vi "HW Display Loop Processor.vi"(4 "error in (no error)":errorcluster) -> (0 "error out":errorcluster, 1 "Tx Stat":T1, 2 "TxPower":dbl[](array[numeric]) format="%.2f", 3 "TxOn":bool[](array[boolean]))   [LabVIEW 2011]
uses:
  API/Controls/PIM.API.Command.Unique.ctl
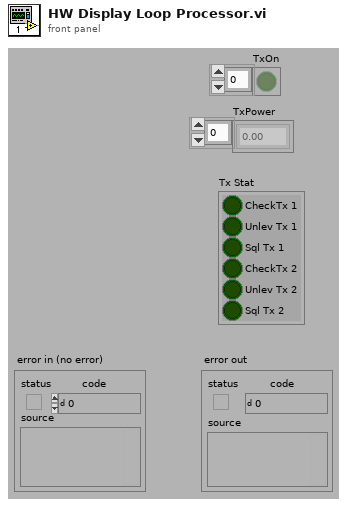
[diagram p1: front panel]
types:
  T1 = cluster{"CheckTx 1":bool, "Unlev Tx 1":bool, "Sql Tx 1":bool, "CheckTx 2":bool, "Unlev Tx 2":bool, "Sql Tx 2":bool}
  T2 = typedef "PIM.API.Command.Unique.ctl" = cluster{"#attributes":cluster{"Action":string}, "Double":dbl[], "Integer":i32[], "Boolean":bool[], "String":string[]}
  T3 = typedef "PIM.API.Response.Unique.ctl" = cluster{"#attributes":cluster{"Action":string, "Units":string}, "Double":dbl[], "Integer":i32[], "Boolean":bool[], "String":string[], "Sample":T4[], "Status":cluster{"#attributes":cluster{"Error":bool, "Code":i32}, "Message":string}[]}
  T4 = typedef "PIM.API.Response.Samples.ctl" = cluster{"TX1":cluster{"#attributes":cluster{"Frequency":dbl, "Power_dBm":dbl, "Power_Watts":dbl, "CheckTx":bool, "Unleveled":bool, "Squelched":bool, "Temperature":dbl, "ToneOn":bool}}, "TX2":cluster{"#attributes":cluster{"Frequency":dbl, "Power_dBm":dbl, "Power_Watts":dbl, "CheckTx":bool, "Unleveled":bool, "Squelched":bool, "Temperature":dbl, "ToneOn":bool}}, "IM":cluster{"#attributes":cluster{"Frequency":dbl, "Power_dBm":dbl, "PeakPower_dBm":dbl, "Power_dBc":dbl, "PeakPower_dBc":dbl, "IM_Order":u8, "IM Overload":bool}}[], "#attributes":cluster{"Count":u32, "Total":u32, "Finished?":bool, "Sweep Leg":T5, "F1":dbl, "F2":dbl, "FStep":dbl}}
  T5 = typedef "iQA Sweep Behavior.ctl" = enum16{"F2Down", "F1Up", "RxMultiIM"}
  T6 = cluster{"#attributes":cluster{"Error":bool, "Code":i32}, "Message":string}[]
  T7 = cluster{"#attributes":cluster{"Error":bool, "Code":i32}, "Message":string}
  T8 = cluster{"Boolean[0]":bool, "Boolean[1]":bool, "Boolean[2]":bool, "Boolean[3]":bool, "Boolean[4]":bool, "Boolean[5]":bool}
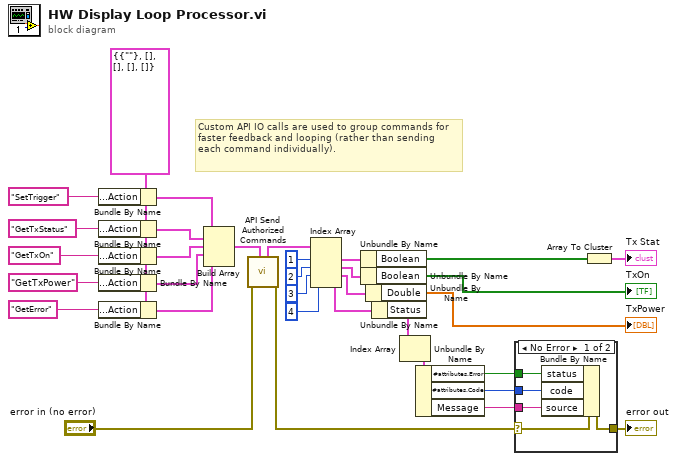
[diagram p0: block diagram]
diagram:
  w13 = T2 {"#attributes"={"Action"=""}, "Double"=[], "Integer"=[], "Boolean"=[], "String"=[]}
  # "Custom API IO calls are used to group commands for faster feedback and looping (rather than sending each command individually)."
  n1 = Bundle By Name(cluster=w13, "#attributes.Action"="SetTrigger") -> (w29:T2)
  n2 = Bundle By Name(cluster=w13, "#attributes.Action"="GetTxStatus") -> (w28:T2)
  n3 = Bundle By Name(cluster=w13, "#attributes.Action"="GetTxOn") -> (w27:T2)
  n4 = Bundle By Name(cluster=w13, "#attributes.Action"="GetTxPower") -> (w26:T2)
  n5 = Bundle By Name(cluster=w13, "#attributes.Action"="GetError") -> (w12:T2)
  n6 = Build Array(w29, w28, w27, w26, w12) -> (w2:T2[])
  n7 = call "API Send Authorized Commands.vi"("Commands"=w2, "error in (no error)"="error in (no error)") -> ("error out"=w3:errorcluster, "Responses"=w1:T3[])  [unwired: 7 in, 1 out]
  n8 = Index Array(array=w1, index #1=1 ("index"), index #2=2 ("index"), index #3=3 ("index"), index #4=4 ("index")) -> (element #1=w21:T3, element #2=w20:T3, element #3=w22:T3, element #4=w10:T3)
  n9 = Unbundle By Name(w21) -> ("Boolean"=w18:bool[])
  n10 = Unbundle By Name(w20) -> ("Boolean"=→"TxOn":bool[])
  n11 = Unbundle By Name(w22) -> ("Double"=→"TxPower":dbl[])
  n12 = Unbundle By Name(w10) -> ("Status"=w9:T6)
  n13 = Index Array(array=w9) -> (element=w8:T7)  [unwired: 1 in]
  n14 = Unbundle By Name(w8) -> ("#attributes.Error"=w7:bool, "#attributes.Code"=w6:i32, "Message"=w5:string)
  n15 = case shown="No Error" w3 {
    selector: w3 -> [w34 w39]
    tunnel: w7 -> [w38 _]
    tunnel: w6 -> [w37 _]
    tunnel: w5 -> [w36 _]
    tunnel: [w35 w39] -> w4
    frame No Error {
      n16 = Bundle By Name(cluster=w34, "status"=w38, "code"=w37, "source"=w36) -> (w35:errorcluster)
    }
    frame Error {
    }
  }
  "error out" <- w4
  n17 = Array To Cluster(array=w18) -> (cluster=→"Tx Stat":T8)
